vi "Script WireThroughs (XML).vi"(8 "WireThrough Terminal Names":T3, 11 "IDM Descriptor Array In":T1) -> (3 "Generated XML":string)   [LabVIEW 2021]
uses:
  <vilib>/myRIO/Common/Express VI Framework/typedefs/WireThrough Terminal Names.ctl
  <vilib>/myRIO/Common/Express VI Framework/typedefs/Instrument Driver Method Descriptor Array.ctl
  <vilib>/myRIO/Common/Express VI Framework/typedefs/Instrument Driver Method Descriptor.ctl
  <vilib>/myRIO/Common/Express VI Framework/typedefs/Create FP Controls Actions.ctl
  <vilib>/_script/XML Scripting/XML Script - Wire (BD).vi
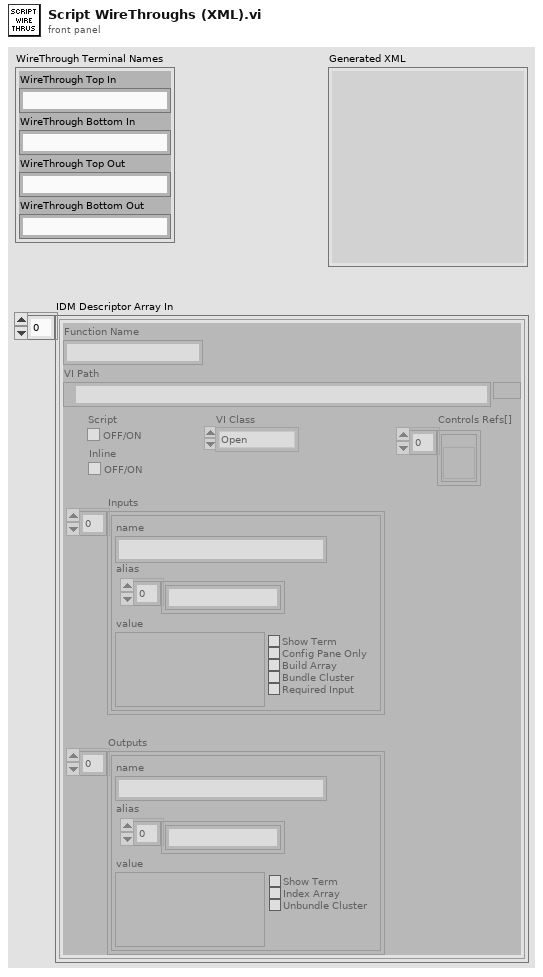
[diagram p1: front panel]
types:
  T1 = typedef "Instrument Driver Method Descriptor Array.ctl" = T2[]
  T2 = typedef "Instrument Driver Method Descriptor.ctl" = cluster{"Function Name":string, "VI Path":path, "Script":bool, "Inputs":cluster{"name":string, "value":variant, "Config Pane Only":bool, "Build Array":bool, "Bundle Cluster":bool, "Show Term":bool, "alias":string[], "Required Input":bool}[], "Outputs":cluster{"name":string, "value":variant, "Show Term":bool, "Index Array":bool, "Unbundle Cluster":bool, "alias":string[]}[], "VI Class":enum16{"Open", "Configure", "Data", "Manage", "Close"}, "Controls Refs[]":refnum<vi>[], "Inline":bool}
  T3 = typedef "WireThrough Terminal Names.ctl" = cluster{"WireThrough Top In":string, "WireThrough Bottom In":string, "WireThrough Top Out":string, "WireThrough Bottom Out":string}
  T4 = typedef "Create FP Controls Actions.ctl" = enum16{"Create Control", "Create Indicator", "Create Constant", "Build Array", "Index Array", "Create Error In", "Create Error Out", "Bundle Cluster", "Unbundle Cluster"}
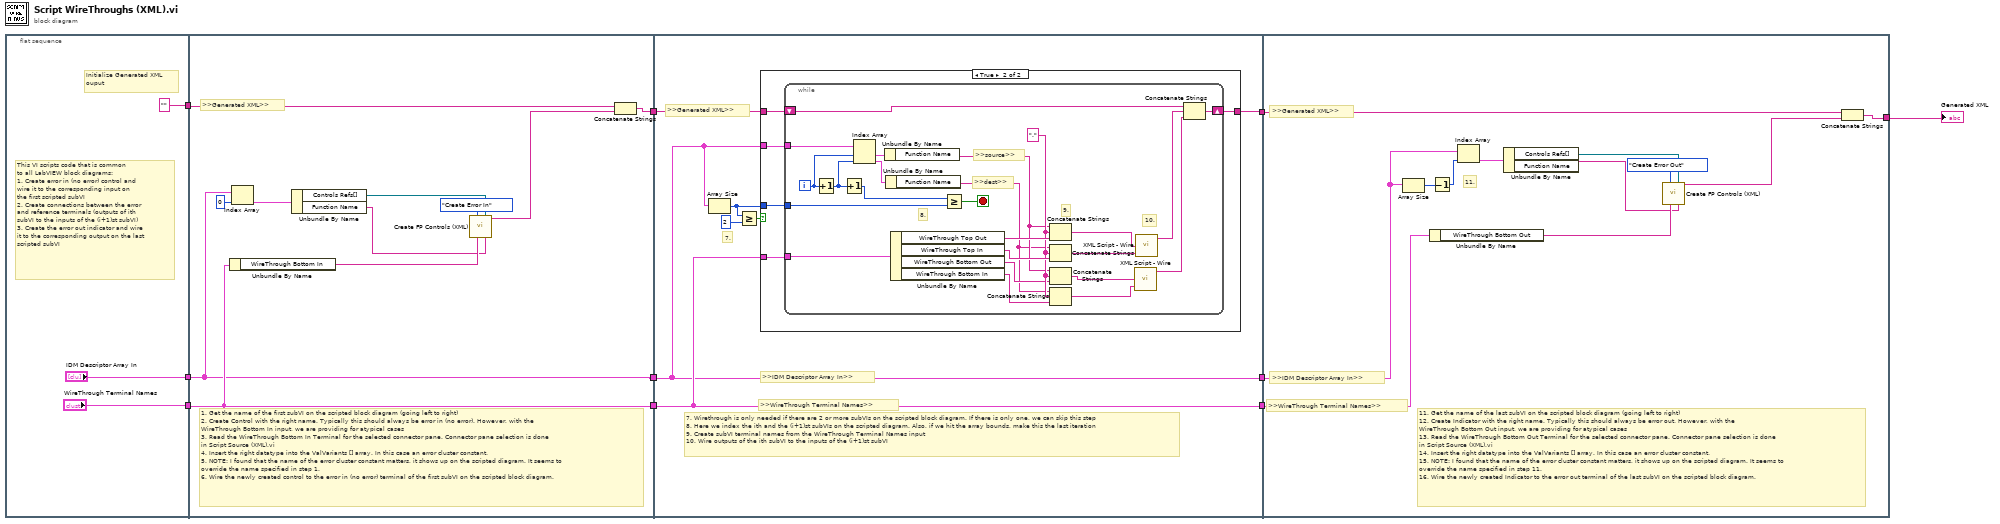
[diagram p0: block diagram]
diagram:
  n1 = flat-sequence {
    tunnel: [""] -> w10
    tunnel: ["WireThrough Terminal Names"] -> w9
    tunnel: ["IDM Descriptor Array In"] -> w3
    tunnel: w10 -> [w22]
    tunnel: w9 -> [w18]
    tunnel: [w21] -> w8
    tunnel: [w18] -> w5
    tunnel: w3 -> [w17]
    tunnel: [w17] -> w2
    tunnel: w8 -> [w28]
    tunnel: [w27] -> w7
    tunnel: w5 -> [w26]
    tunnel: [w26] -> w4
    tunnel: w2 -> [w25]
    tunnel: [w25] -> w1
    tunnel: [w73] -> w6
    tunnel: w1 -> [w65]
    tunnel: w4 -> [w67]
    tunnel: w7 -> [w68]
    frame #0 {
      # "This VI scripts code that is common\nto all LabVIEW block diagrams:\n1. Create error in (no error) control and \nwire it to the corresponding input on\nthe first scripted subVI\n2. Create connections between the error\nand reference terminals (outputs of ith \nsubVI to the inputs of the (i+1)st subVI)\n3. Create the error out indicator and wire\nit to the corresponding output on the last\nscripted subVI"
      # "Initialize Generated XML\nouput"
    }
    frame #1 {
      # "1. Get the name of the first subVI on the scripted block diagram (going left to right)\n2. Create Control with the right name. Typically this should always be error in (no error). However, with the \nWireThrough Bottom In input, we are providing for atypical cases\n3. Read the WireThrough Bottom In Terminal for the selected connector pane. Connector pane selection is done\nin Script Source (XML).vi\n4. Insert the right datatype into the ValVariants [] array. In this case an error cluster constant.\n5. NOTE: I found that the name of the error cluster constant matters, it shows up on the scripted diagram. It seems to\noverride the name specified in step 1.\n6. Wire the newly created control to the error in (no error) terminal of the first subVI on the scripted block diagram."
      # ">>Generated XML>>"
      n2 = Unbundle By Name(w18) -> ("WireThrough Bottom In"=w19:string)
      n3 = Index Array(array=w17, index=0) -> (element=w23:T2)
      n4 = Unbundle By Name(w23) -> ("Controls Refs[]"=w15:refnum<vi>[], "Function Name"=w16:string)
      n5 = call <vilib>:"Create FP Controls (XML).vi"("Action"=Create_FP_Controls_Actions."Create Error In", "Controls Refs[]"=w15, "Terminal Name"=w19, "Function Name"=w16) -> ("Generated XML"=w20:string)  [unwired: 8 in, 3 out]
      n6 = Concatenate Strings(w22, w20) -> (w21:string)
    }
    frame #2 {
      # "7. Wirethrough is only needed if there are 2 or more subVIs on the scripted block diagram. If there is only one, we can skip this step\n8. Here we index the ith and the (i+1)st subVIs on the scripted diagram. Also, if we hit the array bounds, make this the last iteration\n9. Create subVI terminal names from the WireThrough Terminal Names input\n10. Wire outputs of the ith subVI to the inputs of the (i+1)st subVI"
      # "7."
      # ">>Generated XML>>"
      # ">>WireThrough Terminal Names>>"
      # ">>IDM Descriptor Array In>>"
      n7 = Array Size(array=w25) -> (size(s)=w31:i32)
      n8 = Greater Or Equal?(x=w31, y=2) -> (x >= y?=w29:bool)
      n9 = case shown="True" w29 {
        tunnel: w28 -> [w32 w37]
        tunnel: [w32 w36] -> w27
        tunnel: w26 -> [_ w35]
        tunnel: w25 -> [_ w34]
        tunnel: w31 -> [_ w33]
        frame False {
        }
        frame True {
          n10 = while {
            tunnel: w34 -> [w61]
            tunnel: w35 -> [w59]
            shift-right: [w48] -> w36
            shift-left: w37 -> [w47]
            tunnel: w33 -> [w40]
            i -> [w46]
            stop <- w41 stop-if-true
            w55 = "." ("string")
            # "10."
            # "9."
            # "8."
            # ">>dest>>"
            # ">>source>>"
            n11 = Increment(x=w46) -> (x+1=w45:i32)
            n12 = Increment(x=w45) -> (x+1=w44:i32)
            n13 = Index Array(array=w61, index #1=w46, index #2=w45) -> (element #1=w42:T2, element #2=w43:T2)
            n14 = Unbundle By Name(w42) -> ("Function Name"=w39:string)
            n15 = Unbundle By Name(w43) -> ("Function Name"=w38:string)
            n16 = Unbundle By Name(w59) -> ("WireThrough Top Out"=w60:string, "WireThrough Top In"=w58:string, "WireThrough Bottom Out"=w54:string, "WireThrough Bottom In"=w53:string)
            n17 = Greater Or Equal?(x=w44, y=w40) -> (x >= y?=w41:bool)
            n18 = Concatenate Strings(w39, w55, w60) -> (w57:string)
            n19 = Concatenate Strings(w38, w55, w58) -> (w56:string)
            n20 = Concatenate Strings(w39, w55, w54) -> (w52:string)
            n21 = Concatenate Strings(w38, w55, w53) -> (w51:string)
            n22 = call-poly <vilib>:"XML Script - Wire.vi"("destination"=w51, "source"=w52) -> ("XML Script Command - Wire"=w49:string)  [unwired: 1 in, 2 out]
            n23 = call-poly <vilib>:"XML Script - Wire.vi"("destination"=w56, "source"=w57) -> ("XML Script Command - Wire"=w50:string)  [unwired: 1 in, 2 out]
            n24 = Concatenate Strings(w47, w50, w49) -> (w48:string)
          }
        }
      }
    }
    frame #3 {
      # "11."
      # "11. Get the name of the last subVI on the scripted block diagram (going left to right)\n12. Create Indicator with the right name. Typically this should always be error out. However, with the \nWireThrough Bottom Out input, we are providing for atypical cases\n13. Read the WireThrough Bottom Out Terminal for the selected connector pane. Connector pane selection is done\nin Script Source (XML).vi\n14. Insert the right datatype into the ValVariants [] array. In this case an error cluster constant.\n15. NOTE: I found that the name of the error cluster constant matters, it shows up on the scripted diagram. It seems to\noverride the name specified in step 11.\n16. Wire the newly created Indicator to the error out terminal of the last subVI on the scripted block diagram."
      # ">>Generated XML>>"
      # ">>WireThrough Terminal Names>>"
      # ">>IDM Descriptor Array In>>"
      n25 = Array Size(array=w65) -> (size(s)=w71:i32)
      n26 = Unbundle By Name(w67) -> ("WireThrough Bottom Out"=w66:string)
      n27 = Decrement(x=w71) -> (x-1=w72:i32)
      n28 = Index Array(array=w65, index=w72) -> (element=w70:T2)
      n29 = Unbundle By Name(w70) -> ("Controls Refs[]"=w63:refnum<vi>[], "Function Name"=w64:string)
      n30 = call <vilib>:"Create FP Controls (XML).vi"("Action"=Create_FP_Controls_Actions."Create Error Out", "Controls Refs[]"=w63, "Terminal Name"=w66, "Function Name"=w64) -> ("Generated XML"=w69:string)  [unwired: 8 in, 3 out]
      n31 = Concatenate Strings(w68, w69) -> (w73:string)
    }
  }
  "Generated XML" <- w6
